vi "Write tx transfer settings.vi"(8 "error in (no error)":errorcluster, 10 "tx transfer settings":T1, 11 "UDPlog Transfer Tx Configuration in":refnum<class "UDPlog Transfer Tx Configuration.lvclass">) -> (0 "error out":errorcluster, 3 "UDPlog Transfer Tx Configuration out":refnum<class "UDPlog Transfer Tx Configuration.lvclass">)   [LabVIEW 2023, in "UDPlog.lvlib" / "UDPlog Transfer Tx Configuration.lvclass"]
uses:
  UDPlog Transfer Tx Configuration.lvclass
  UDPlog Transfer Tx Configuration.lvclass/UDPlog Transfer Tx Configuration.ctl
  Tx Transfer Settings.ctl
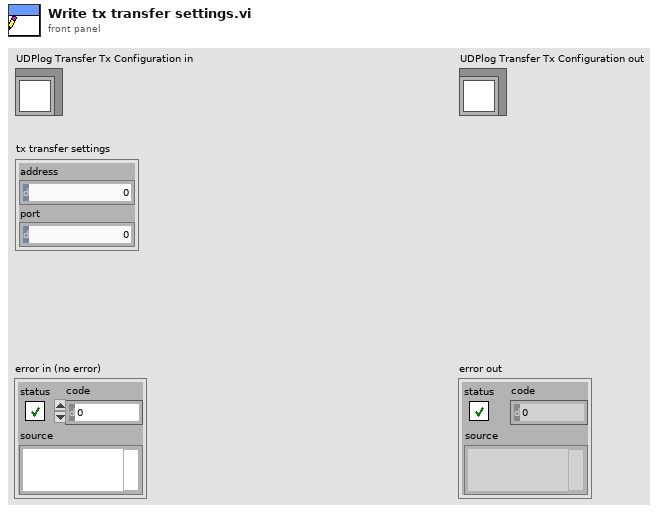
[diagram p1: front panel]
types:
  T1 = typedef "Tx Transfer Settings.ctl" = cluster{"address":u32, "port":u16}
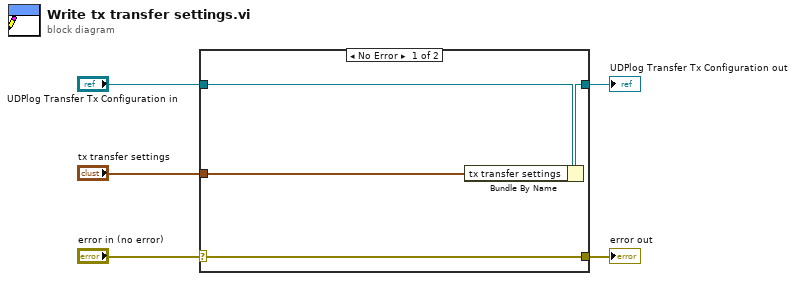
[diagram p0: block diagram]
diagram:
  n1 = case shown="No Error" "error in (no error)" {
    selector: "error in (no error)" -> [w9 w10]
    tunnel: [w9 w10] -> w4
    tunnel: [w7 w11] -> w2
    tunnel: "UDPlog Transfer Tx Configuration in" -> [w8 w11]
    tunnel: "tx transfer settings" -> [w6 _]
    frame No Error {
      n2 = Bundle By Name(cluster=w8, "tx transfer settings"=w6) -> (w7:refnum<class "UDPlog Transfer Tx Configuration.lvclass">)
    }
    frame Error {
    }
  }
  "error out" <- w4
  "UDPlog Transfer Tx Configuration out" <- w2
